vi "MainCircuit.vi"() -> ()   [LabVIEW 2014]
uses:
  <vilib>/myRIO/Instrument Drivers/Onboard Devices/Accelerometer/typedefs/Accelerometer Reference.ctl
  <vilib>/myRIO/Common/Instrument Driver Framework/Utilities/typedefs/myRIO Generic Hardware Reference.ctl
  <vilib>/myRIO/Common/Instrument Driver Framework/Utilities/typedefs/Hardware Version Enum.ctl
  <vilib>/myRIO/Common/Instrument Driver Framework/Utilities/typedefs/myRIO v1.0 Reference.ctl
  <vilib>/myRIO/Common/Instrument Driver Framework/Utilities/typedefs/Generic FPGA Reference.ctl
  <vilib>/myRIO/Common/Instrument Driver Framework/myRIO v1.0/Accelerometer/typedefs/Accelerometer Channels List.ctl
  <vilib>/myRIO/Common/Instrument Driver Framework/myRIO v1.0/Accelerometer/typedefs/Accelerometer Channels Enum.ctl
  <vilib>/userdefined/High Color/nirio_resource_hc.ctl
  <vilib>/myRIO/Common/Instrument Driver Framework/Utilities/vis/Is FPGA Ref Available.vi
  <vilib>/myRIO/Common/Instrument Driver Framework/myRIO v1.0/Accelerometer/vis/myRIO v1.1 Open Accelerometer.vi
  <vilib>/myRIO/Instrument Drivers/Onboard Devices/Accelerometer/vis/Read.vi
  <vilib>/myRIO/Common/Instrument Driver Framework/Utilities/vis/Validate Channels.vi
  <vilib>/myRIO/Common/Instrument Driver Framework/myRIO v1.0/Accelerometer/vis/myRIO v1.0 Reserve Accelerometer.vi
  <vilib>/myRIO/Common/Instrument Driver Framework/myRIO v1.0/UART/vis/myRIO v1.0 Close UART.vi
  <vilib>/myRIO/Common/Instrument Driver Framework/myRIO v1.0/Resource Manager/vis/myRIO v1.0 Reserve Channel List.vi
  <vilib>/myRIO/Common/Instrument Driver Framework/myRIO v1.0/Accelerometer/vis/myRIO v1.0 Build MUX Configuration Accelerometer.vi
  <vilib>/myRIO/Common/Instrument Driver Framework/myRIO v1.0/Resource Manager/vis/myRIO v1.0 Reserve Channel.vi
  <vilib>/myRIO/Common/Instrument Driver Framework/myRIO v1.0/Resource Manager/vis/myRIO v1.0 Unreserve Channel.vi
  <vilib>/myRIO/Common/Instrument Driver Framework/myRIO v1.0/Resource Manager/vis/myRIO v1.0 Build Mutex Name.vi
  <vilib>/Utility/VariantDataType/GetNumericInfo.vi
  <vilib>/Utility/error.llb/Error Cluster From Error Code.vi
  <vilib>/myRIO/Common/Instrument Driver Framework/myRIO v1.0/myRIO v1.1 Open.vi
  <vilib>/myRIO/Common/Instrument Driver Framework/myRIO v1.0/Accelerometer/vis/myRIO v1.0 Get Scaling Constant Accelerometer.vi
  <vilib>/myRIO/Common/Instrument Driver Framework/Utilities/vis/IO Manager.vi
  <vilib>/myRIO/Common/Instrument Driver Framework/Utilities/vis/Configuration Manager.vi
  <vilib>/myRIO/Common/Instrument Driver Framework/myRIO v1.0/myRIO v1.0 Close.vi
  <vilib>/myRIO/Common/Instrument Driver Framework/myRIO v1.0/Accelerometer/vis/myRIO v1.0 Read Accelerometer.vi
  <vilib>/myRIO/Common/Instrument Driver Framework/Utilities/vis/FPGA Ref Manager.vi
  <vilib>/myRIO/Common/Instrument Driver Framework/myRIO v1.0/myRIO v1.0 Reset FPGA.vi
  <vilib>/myRIO/Common/Instrument Driver Framework/myRIO v1.0/IRQ/vis/myRIO v1.0 IRQ Info FGV.vi
  <vilib>/myRIO/Common/Instrument Driver Framework/myRIO v1.0/IRQ/vis/myRIO v1.0 Timer IRQ Info FGV.vi
  <vilib>/myRIO/Common/Instrument Driver Framework/myRIO v1.0/IRQ/vis/myRIO v1.0 ISR Agent.vi
  <vilib>/myRIO/Express VI/Onboard Devices/Accelerometer/Accelerometer Express VI.xnode
  <vilib>/myRIO/Instrument Drivers/Onboard Devices/Accelerometer/vis/myRIO Accelerometer Open.xnode
  <vilib>/myRIO/Instrument Drivers/Onboard Devices/Accelerometer/Accelerometer.lvlib
  <vilib>/myRIO/Instrument Drivers/Utilities/Utilities.lvlib
panel:
  in  "Learning Factor":dbl
  in  "ExpectedZ":dbl
  in  "ExpectedY":dbl
  in  "ExpectedX":dbl
  out "h3":dbl
  out "h2":dbl
  out "h1":dbl
  out "Z":dbl
  out "X":dbl
  out "Y":dbl
  out "error out":errorcluster
  out "Waveform Chart":T1(graph)
  in  "stop":bool
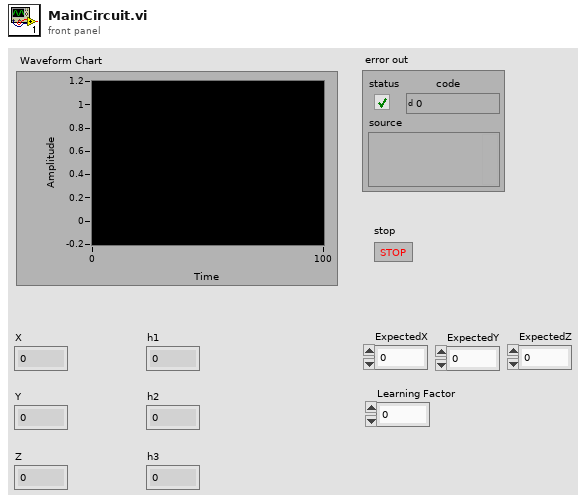
[diagram p1: front panel]
types:
  T1 = cluster{"X-Axis":dbl, "Y-Axis":dbl, "Z-Axis":dbl}
  T2 = typedef "Accelerometer.lvlib/Accelerometer Reference.ctl" = cluster{"myRIO Reference":T3, "Accelerometer Channels List":T7, "LSB Weight":dbl}
  T3 = typedef "myRIO Generic Hardware Reference.ctl" = cluster{"myRIO Model":T4, "myRIO Hardware Reference":T5}
  T4 = typedef "Hardware Version Enum.ctl" = enum16{"Unknown", "myRIO-1900", "myRIO-1950"}
  T5 = typedef "myRIO v1.0 Reference.ctl" = cluster{"Generic FPGA Reference":T6, "Allow multiple opens":bool}
  T6 = typedef "Generic FPGA Reference.ctl" = refnum<k20>
  T7 = typedef "Accelerometer Channels List.ctl" = T8[]
  T8 = typedef "Accelerometer Channels Enum.ctl" = enum16{"Not Connected", "X-Axis", "Y-Axis", "Z-Axis"}
  T9 = typedef "nirio_resource_hc.ctl" = tag
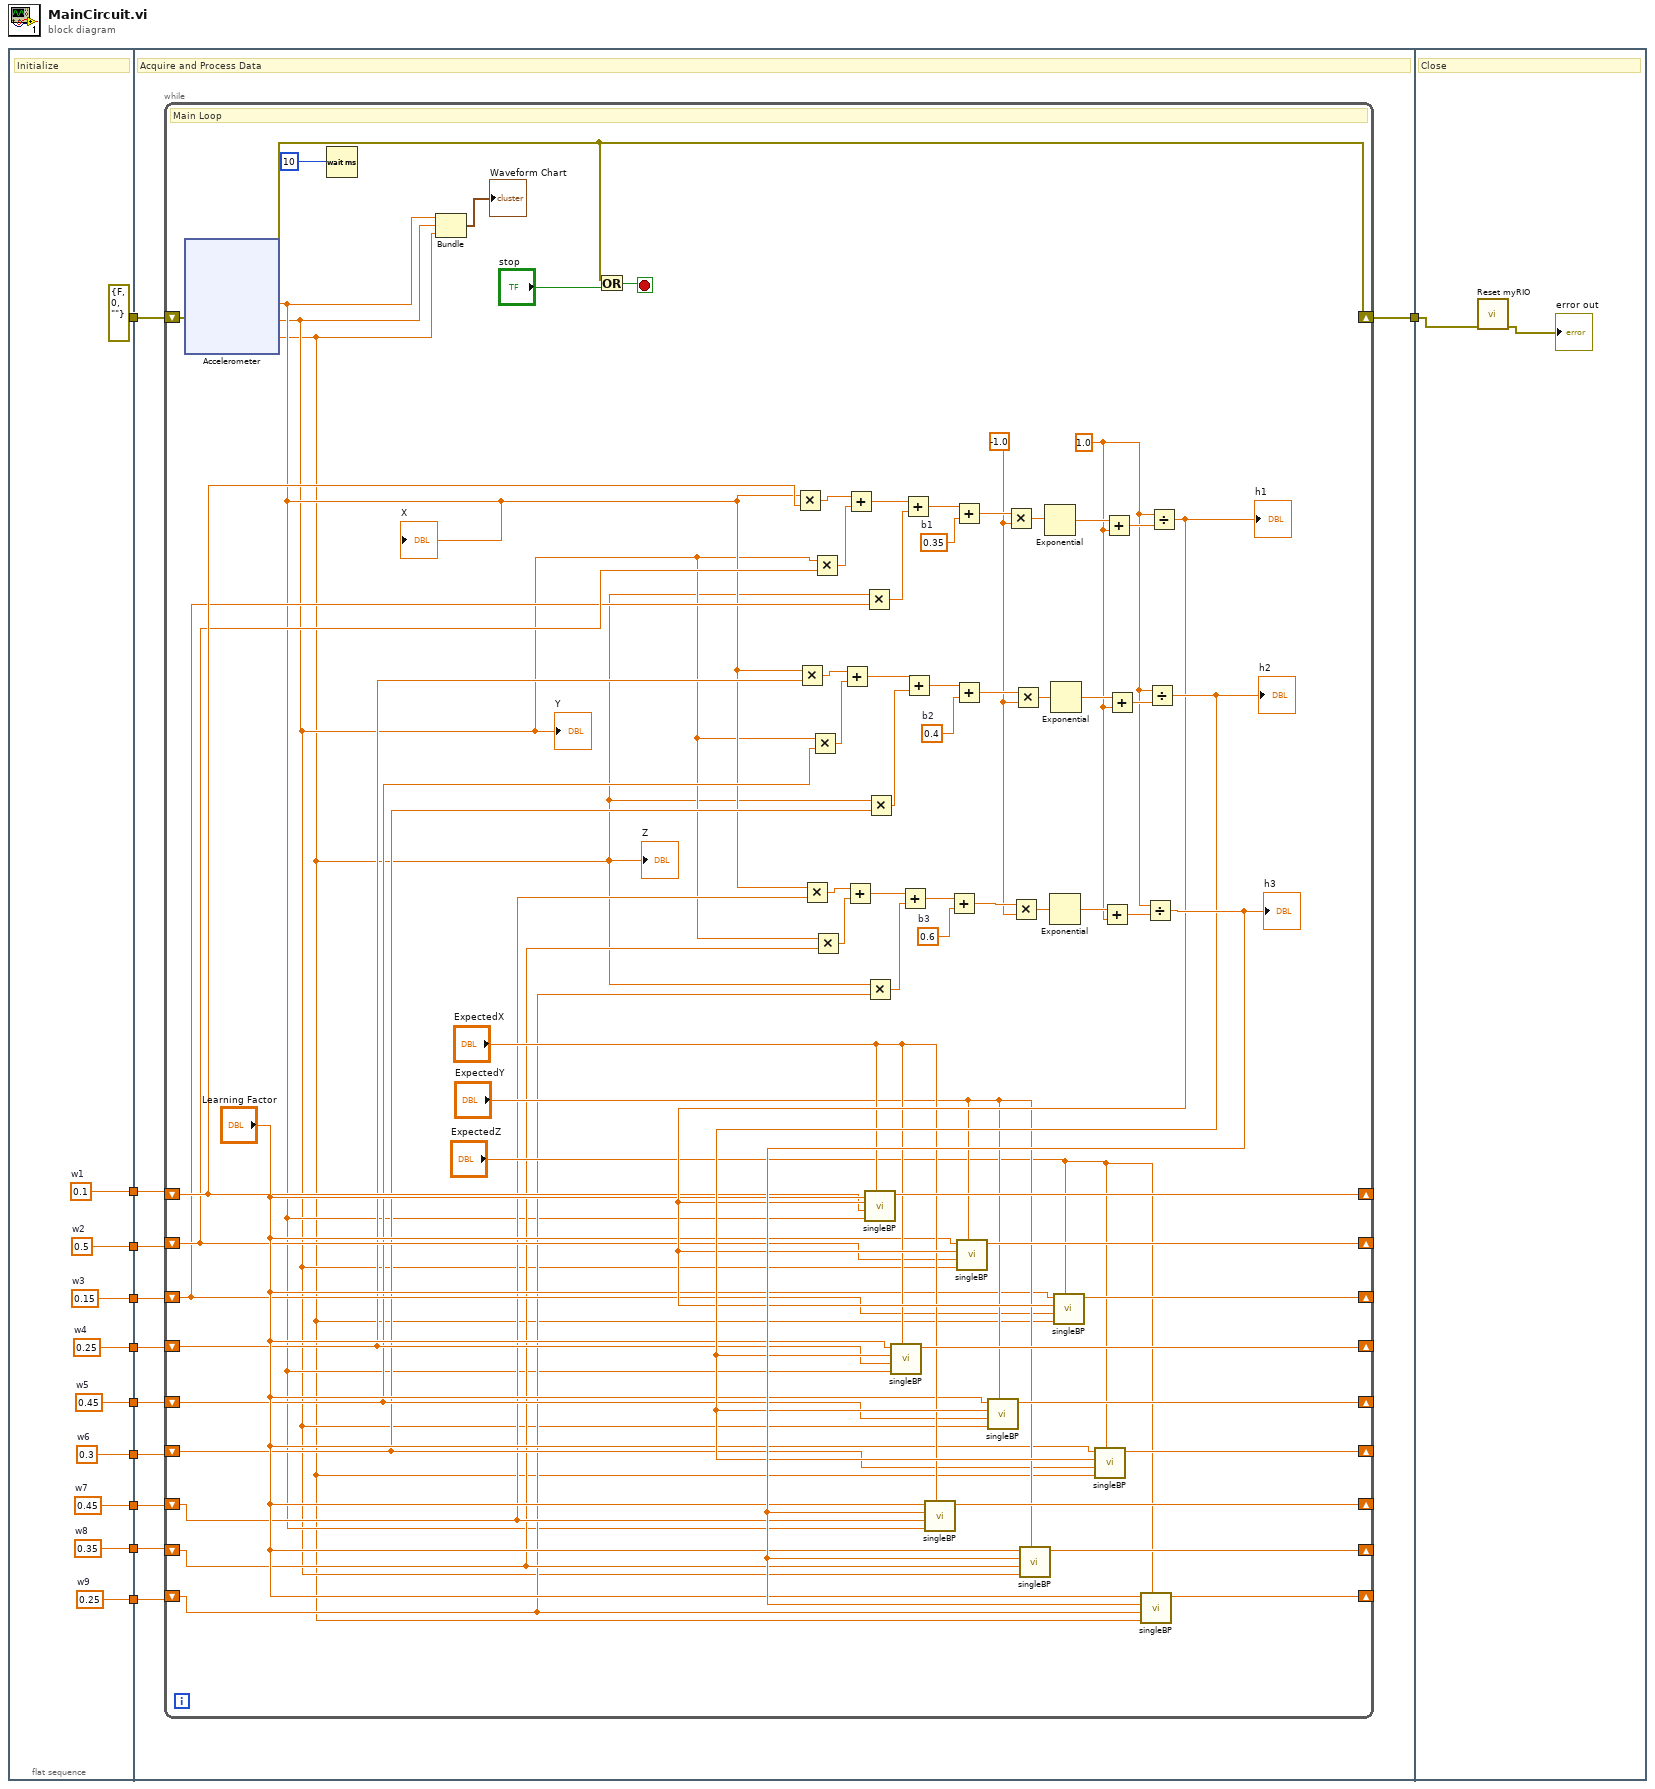
[diagram p0: block diagram]
diagram:
  n1 = flat-sequence {
    tunnel: [errorcluster {"status"=FALSE, "code"=0, "source"=""} ("error out")] -> w10
    tunnel: [w20] -> w9
    tunnel: [w19] -> w8
    tunnel: [w18] -> w7
    tunnel: [w17] -> w6
    tunnel: [w16] -> w5
    tunnel: [w15] -> w4
    tunnel: [w14] -> w3
    tunnel: [w13] -> w2
    tunnel: [w12] -> w1
    tunnel: [w32] -> w11
    tunnel: w10 -> [w31]
    tunnel: w9 -> [w30]
    tunnel: w8 -> [w29]
    tunnel: w7 -> [w28]
    tunnel: w6 -> [w27]
    tunnel: w5 -> [w26]
    tunnel: w4 -> [w25]
    tunnel: w3 -> [w24]
    tunnel: w2 -> [w23]
    tunnel: w1 -> [w22]
    tunnel: w11 -> [w139]
    frame #0 {
      w12 = 0.25  # w9
      w13 = 0.35  # w8
      w14 = 0.45  # w7
      w15 = 0.3  # w6
      w16 = 0.45  # w5
      w17 = 0.25  # w4
      w18 = 0.15  # w3
      w19 = 0.5  # w2
      w20 = 0.1  # w1
      # "Initialize"
    }
    frame #1 {
      # "Acquire and Process Data"
      n2 = while {
        shift-right: [w95] -> w32
        shift-left: w31 -> [w94]
        shift-right: [w52] -> _
        shift-left: w30 -> [w44]
        shift-right: [w53] -> _
        shift-left: w29 -> [w43]
        shift-right: [w54] -> _
        shift-left: w28 -> [w42]
        shift-right: [w55] -> _
        shift-left: w27 -> [w41]
        shift-right: [w56] -> _
        shift-left: w26 -> [w40]
        shift-right: [w57] -> _
        shift-left: w25 -> [w39]
        shift-right: [w58] -> _
        shift-left: w24 -> [w38]
        shift-right: [w59] -> _
        shift-left: w23 -> [w37]
        shift-right: [w60] -> _
        shift-left: w22 -> [w36]
        stop <- w93 stop-if-true
        w61 = 1.0
        w71 = -1.0
        w75 = 0.6  # b3
        w76 = 0.4  # b2
        w77 = 0.35  # b1
        # "Main Loop"
        n3 = xnode "Accelerometer"("error in (no error)"=w94) -> ("X-Axis"=w35:dbl, "Y-Axis"=w34:dbl, "Z-Axis"=w33:dbl, "error out"=w95:errorcluster)
        "Y" <- w34
        "X" <- w35
        "Z" <- w33
        n4 = Wait (ms)(milliseconds to wait=10) -> ()  [unwired: 1 out]
        n5 = Bundle "Bundle"("X-Axis"=w35, "Y-Axis"=w34, "Z-Axis"=w33) -> (→"Waveform Chart":T1)  [unwired: 1 in]
        n6 = Or(x=w95, y="stop") -> (x .or. y?=w93:bool)
        n7 = Multiply(x=w35, y=w44) -> (x*y=w92:dbl)
        n8 = Multiply(x=w35, y=w41) -> (x*y=w91:dbl)
        n9 = Multiply(x=w35, y=w38) -> (x*y=w90:dbl)
        n10 = Multiply(x=w34, y=w40) -> (x*y=w88:dbl)
        n11 = Multiply(x=w34, y=w43) -> (x*y=w89:dbl)
        n12 = Multiply(x=w34, y=w37) -> (x*y=w87:dbl)
        n13 = Add(x=w91, y=w88) -> (x+y=w86:dbl)
        n14 = Add(x=w90, y=w87) -> (x+y=w84:dbl)
        n15 = Add(x=w92, y=w89) -> (x+y=w85:dbl)
        n16 = Multiply(x=w33, y=w42) -> (x*y=w81:dbl)
        n17 = Multiply(x=w33, y=w36) -> (x*y=w82:dbl)
        n18 = Multiply(x=w33, y=w39) -> (x*y=w83:dbl)
        n19 = Add(x=w84, y=w82) -> (x+y=w78:dbl)
        n20 = Add(x=w85, y=w81) -> (x+y=w80:dbl)
        n21 = Add(x=w86, y=w83) -> (x+y=w79:dbl)
        n22 = Add(x=w78, y=w75) -> (x+y=w74:dbl)
        n23 = Add(x=w80, y=w77) -> (x+y=w72:dbl)
        n24 = Add(x=w79, y=w76) -> (x+y=w73:dbl)
        n25 = Multiply(x=w72, y=w71) -> (x*y=w70:dbl)
        n26 = Multiply(x=w74, y=w71) -> (x*y=w68:dbl)
        n27 = Multiply(x=w73, y=w71) -> (x*y=w69:dbl)
        n28 = Exponential(1:w70) -> (0:w65:dbl)
        n29 = Exponential(1:w68) -> (0:w67:dbl)
        n30 = Exponential(1:w69) -> (0:w66:dbl)
        n31 = Add(x=w67, y=w61) -> (x+y=w62:dbl)
        n32 = Add(x=w65, y=w61) -> (x+y=w64:dbl)
        n33 = Add(x=w66, y=w61) -> (x+y=w63:dbl)
        n34 = Divide(x=w61, y=w62) -> (x/y=w51:dbl)
        "h3" <- w51
        n35 = call "singleBP.vi"("Expected"="ExpectedX", "AccelValue"=w35, "Weight"=w38, "Output"=w51, "LearningFactor"="Learning Factor") -> ("NewWeight"=w58:dbl)  [unwired: 6 in]
        n36 = call "singleBP.vi"("Expected"="ExpectedY", "AccelValue"=w34, "Weight"=w37, "Output"=w51, "LearningFactor"="Learning Factor") -> ("NewWeight"=w59:dbl)  [unwired: 6 in]
        n37 = call "singleBP.vi"("Expected"="ExpectedZ", "AccelValue"=w33, "Weight"=w36, "Output"=w51, "LearningFactor"="Learning Factor") -> ("NewWeight"=w60:dbl)  [unwired: 6 in]
        n38 = Divide(x=w61, y=w63) -> (x/y=w50:dbl)
        "h2" <- w50
        n39 = call "singleBP.vi"("Expected"="ExpectedX", "AccelValue"=w35, "Weight"=w41, "Output"=w50, "LearningFactor"="Learning Factor") -> ("NewWeight"=w55:dbl)  [unwired: 6 in]
        n40 = call "singleBP.vi"("Expected"="ExpectedY", "AccelValue"=w34, "Weight"=w40, "Output"=w50, "LearningFactor"="Learning Factor") -> ("NewWeight"=w56:dbl)  [unwired: 6 in]
        n41 = call "singleBP.vi"("Expected"="ExpectedZ", "AccelValue"=w33, "Weight"=w39, "Output"=w50, "LearningFactor"="Learning Factor") -> ("NewWeight"=w57:dbl)  [unwired: 6 in]
        n42 = Divide(x=w61, y=w64) -> (x/y=w49:dbl)
        "h1" <- w49
        n43 = call "singleBP.vi"("Expected"="ExpectedX", "AccelValue"=w35, "Weight"=w44, "Output"=w49, "LearningFactor"="Learning Factor") -> ("NewWeight"=w52:dbl)  [unwired: 6 in]
        n44 = call "singleBP.vi"("Expected"="ExpectedY", "AccelValue"=w34, "Weight"=w43, "Output"=w49, "LearningFactor"="Learning Factor") -> ("NewWeight"=w53:dbl)  [unwired: 6 in]
        n45 = call "singleBP.vi"("Expected"="ExpectedZ", "AccelValue"=w33, "Weight"=w42, "Output"=w49, "LearningFactor"="Learning Factor") -> ("NewWeight"=w54:dbl)  [unwired: 6 in]
      }
    }
    frame #2 {
      # "Close"
      n46 = call <vilib>:"Reset myRIO.vi"("error in (no error)"=w139) -> ("error out"=→"error out":errorcluster)  [unwired: 10 in]
    }
  }
